vi "init.vi"(8 "error in":errorcluster, 10 "TBM module configuration in":refnum<class "TBM module configuration.lvclass">, 11 "Multiplexer runtime in":refnum<class "Multiplexer runtime.lvclass">) -> (0 "error out":errorcluster, 1 "data allocations":T1, 2 "execution settings":T4, 3 "Multiplexer runtime out":refnum<class "Multiplexer runtime.lvclass">)   [LabVIEW 2021, in "Multiplexer runtime.lvclass"]
doc: "Provides an interface for initializing a module at runtime. While this interface performs no operations, a child should provide an override which may open any necessary references or sessions, allocate necessary memory, and perform any final configuration validataion before providing the full configuration <b>execution data</b> to the calling process."
uses:
  Multiplexer runtime.lvclass
  <vilib>/NI/Tag Bus Module Framework/module configuration/TBM module configuration.lvclass
  <vilib>/NI/Tag Bus Module Framework/runtime/execution settings.ctl
  <vilib>/NI/Tag Bus Module Framework/channel/data tables.ctl
  <vilib>/NI/Tag Bus/dictionary/data dictionary.lvclass
  <vilib>/NI/Tag Bus/dictionary table pair.ctl
  <vilib>/NI/Tag Bus/table/data table.ctl
  configuration/Multiplexer configuration.lvclass
  configuration/Multiplexer configuration.lvclass/Multiplexer configuration.ctl
  Multiplexer runtime.lvclass/Multiplexer runtime.ctl
  configuration/Read Scale.vi
  <vilib>/NI/Tag Bus Module Framework/channel/TBM channel.lvclass
  <vilib>/NI/Tag Bus Module Framework/runtime/TBM module execution interface.lvclass
  <vilib>/NI/Tag Bus/tag bus.lvlib
  <vilib>/NI/Tag Bus/table/data table.lvlib
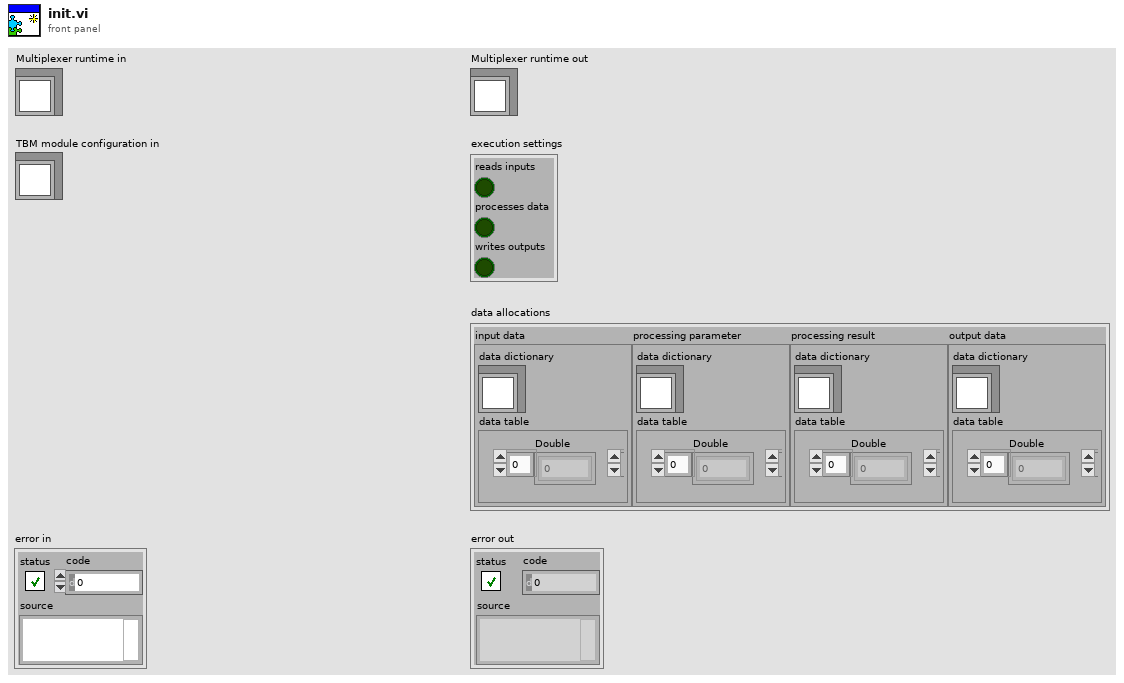
[diagram p1: front panel]
types:
  T1 = typedef "TBM channel.lvclass/data tables.ctl" = cluster{"input data":T2, "processing parameter":T2, "processing result":T2, "output data":T2}
  T2 = typedef "tag bus.lvlib/dictionary table pair.ctl" = cluster{"data dictionary":refnum<class "data dictionary.lvclass">, "data table":T3}
  T3 = typedef "tag bus.lvlib/data table.lvlib/data table.ctl" = cluster{"Double":dbl[], "Single":sgl[], "I64":i64[], "I32":i32[], "I16":i16[], "I8":i8[], "U64":u64[], "U32":u32[], "U16":u16[], "U8":u8[], "Boolean":bool[], "String":string[], "Array of Double":cluster{"DBL Array":dbl[]}[], "Array of Single":cluster{"SGL Array":sgl[]}[], "Array of I64":cluster{"I64 Array":i64[]}[], "Array of I32":cluster{"I32 Array":i32[]}[], "Array of I16":cluster{"I16 Array":i16[]}[], "Array of I8":cluster{"I8 Array":i8[]}[], "Array of U64":cluster{"U64 Array":u64[]}[], "Array of U32":cluster{"U32 Array":u32[]}[], "Array of U16":cluster{"U16 Array":u16[]}[], "Array of U8":cluster{"U8 Array":u8[]}[], "Array of Boolean":cluster{"Boolean Array":bool[]}[], "Array of String":cluster{"String Array":string[]}[]}
  T4 = typedef "TBM module execution interface.lvclass/execution settings.ctl" = cluster{"reads inputs":bool, "processes data":bool, "writes outputs":bool}
  T5 = typedef "Multiplexer runtime.lvclass/Line Mappings.ctl" = cluster{"A":i32, "B":i32, "Select":i32, "Output":i32}
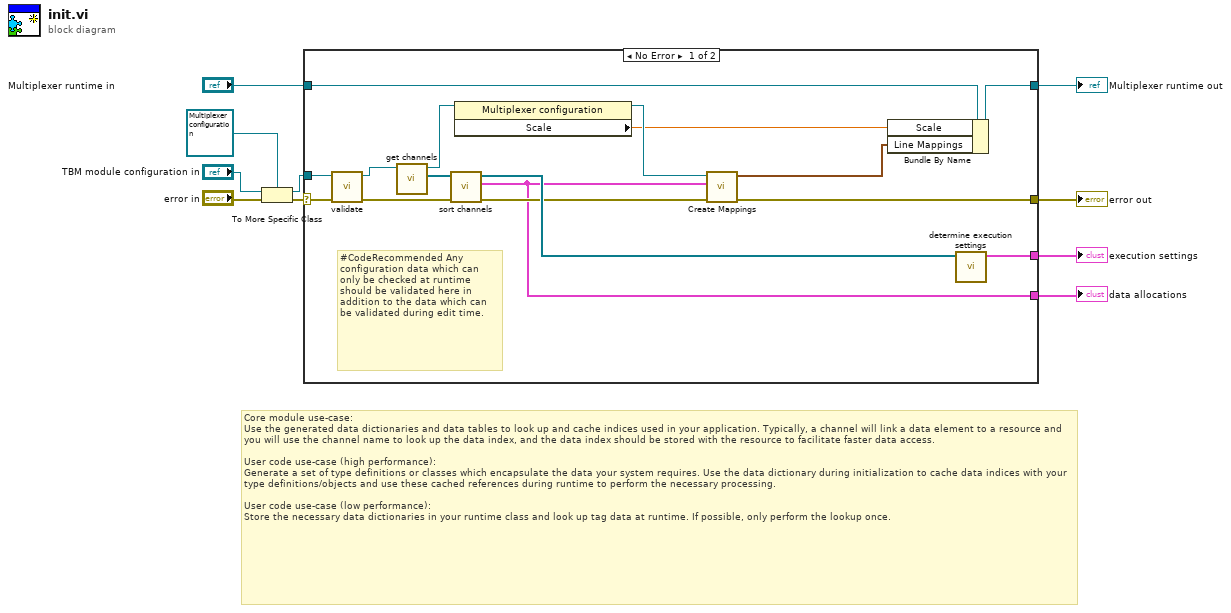
[diagram p0: block diagram]
diagram:
  # "Core module use-case:\nUse the generated data dictionaries and data tables to look up and cache indices used in your application. Typically, a channel will link a data element to a resource and you will use the channel name to look up the data index, and the data index should be stored with the resource to facilitate faster data access.\n\nUser code use-case (high performance):\nGenerate a set of type definitions or classes which encapsulate the data your system requires. Use the data dictionary during initialization to cache data indices with your type definitions/objects and use these cached references during runtime to perform the necessary processing.\n\nUser code use-case (low performance):\nStore the necessary data dictionaries in your runtime class and look up tag data at runtime. If possible, only perform the lookup once."
  n1 = To More Specific Class(target class=refnum<class "Multiplexer configuration.lvclass"> refnum ("Synchronous module configuration"), reference="TBM module configuration in", error in="error in") -> (specific class reference=w9:refnum<class "Multiplexer configuration.lvclass">, error out=w10:errorcluster)
  n2 = case shown="No Error" w10 {
    selector: w10 -> [w22 w27]
    tunnel: w9 -> [w21 _]
    tunnel: "Multiplexer runtime in" -> [w26 w28]
    tunnel: [w13 w28] -> w4
    tunnel: [w15 w27] -> w3
    tunnel: [w14 _] -> w1
    tunnel: [w25 _] -> w2
    frame No Error {
      # "#CodeRecommended Any configuration data which can only be checked at runtime should be validated here in addition to the data which can be validated during edit time."
      n3 = call-dynamic "validate.vi"("error in"=w22, "Multiplexer configuration in"=w21) -> ("error out"=w23:errorcluster, "Multiplexer configuration out"=w20:refnum<class "Multiplexer configuration.lvclass">)  [unwired: 8 in]
      n4 = call-dynamic "get channels.vi"("Multiplexer configuration in"=w20) -> ("channels"=w19:refnum<class "TBM channel.lvclass">[], "Multiplexer configuration out"=w18:refnum<class "Multiplexer configuration.lvclass">)  [unwired: 9 in]
      n5 = call <vilib>:"sort channels.vi"("error in"=w23, "channels in"=w19) -> ("error out"=w16:errorcluster, "data allocations"=w14:T1, "channels out"=w24:refnum<class "TBM channel.lvclass">[])  [unwired: 7 in]
      n6 = property class="Multiplexer configuration"(reference=w18) -> (reference out=w17:refnum<class "Multiplexer configuration.lvclass">, "Scale"=w12:dbl)  [unwired: 1 in, 1 out]
      n7 = call "Create Mappings.vi"("error in (no error)"=w16, "data allocations"=w14, "Multiplexer configuration"=w17) -> ("error out"=w15:errorcluster, "Mappings"=w11:T5[])  [unwired: 7 in]
      n8 = Bundle By Name(cluster=w26, "Scale"=w12, "Line Mappings"=w11) -> (w13:refnum<class "Multiplexer runtime.lvclass">)
      n9 = call <vilib>:"determine execution settings.vi"("channels"=w24) -> ("execution settings"=w25:T4)  [unwired: 10 in]
    }
    frame Error {
    }
  }
  "error out" <- w3
  "Multiplexer runtime out" <- w4
  "execution settings" <- w2
  "data allocations" <- w1
